vi "Coding_morse3.vi"() -> ()   [LabVIEW 2022 SP3]
panel:
  in  "Alphabet":string[][](array[string])=[["a", ".-"], ["b", "-..."], ["c", "-.-."], ["d", "-.."], ["e", "."], ["f", "..-."], ["g", "--."], ["h", "...."], ["i", ".."], ["j", ".---"], ["k", "-.-"], ["l", ".-.."], ["m", "--"], ["n", "-."], ["o", "---"], ["p", ".--."], ["q", "--.-"], ["r", ".-."], ["s", "..."], ["t", "-"], ["u", "..-"], ["v", "...-"], ["w", ".--"], ["x", "-..-"], ["y", "-.--"], ["z", "--.."], ["1", ".----"], ["2", "..---"], ["3", "...--"], ["4", "....-"], ["5", "....."], ["6", "-...."], ["7", "--..."], ["8", "---.."], ["9", "----."], ["0", "-----"], [" ", "space"]]
  in  "Input Words words":string
  out "Whole code":string[](array[string])
  in  "Dit time(ms)":dbl
  in  "Volume":dbl(knob) scale=0.0..100.0
  in  "Frequency":dbl=500.0
  out "Character code remained":i32
  out "current dit/dash time":dbl
  out "String":string
  out "Current code":string
  out "Waiting until next word":bool
  in  "stop":bool
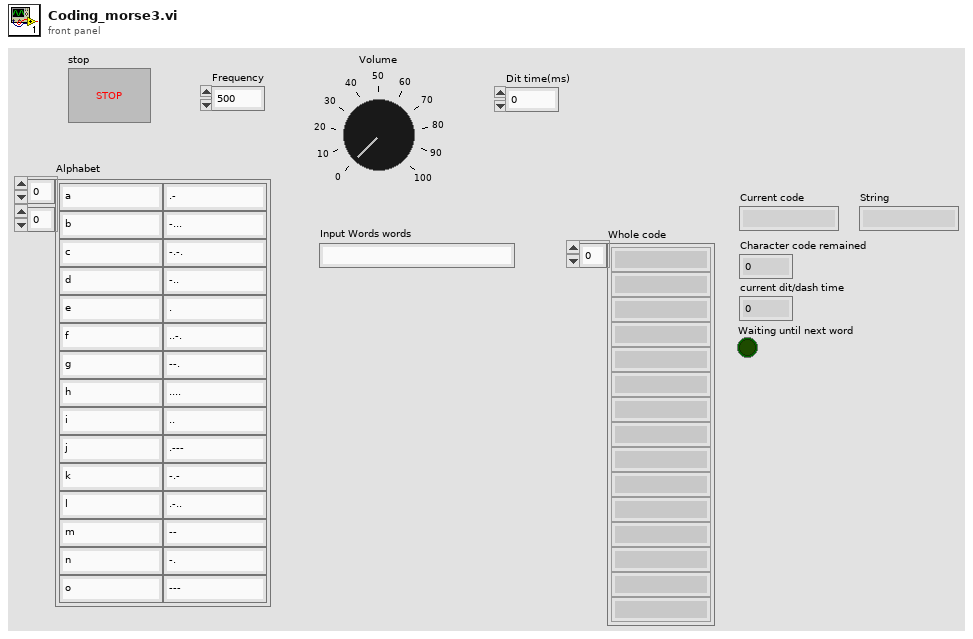
[diagram p1: front panel]
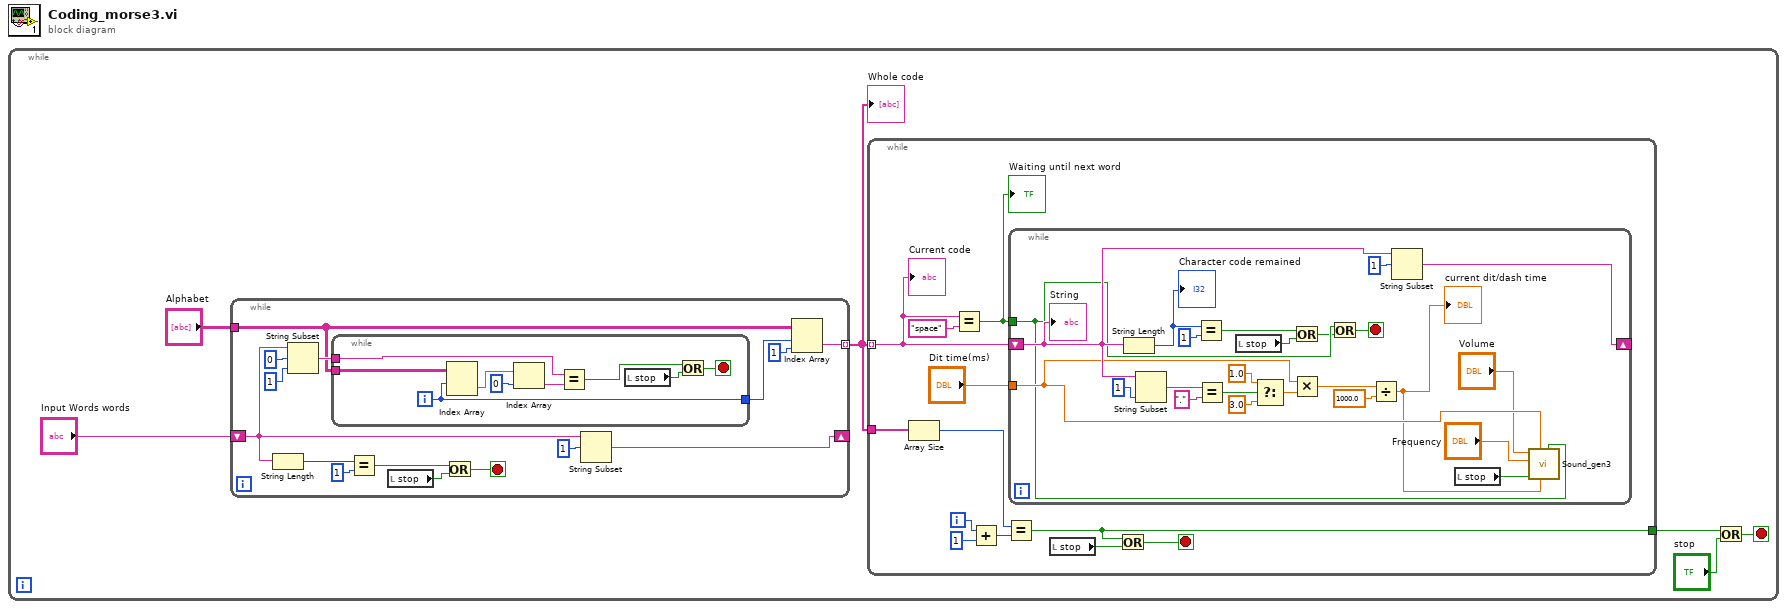
[diagram p0: block diagram]
diagram:
  n1 = while {
    stop <- w1 stop-if-true
    n2 = while {
      shift-right: [w51] -> _
      shift-left: "Input Words words" -> [w52]
      tunnel: "Alphabet" -> [w48]
      tunnel: [w43] -> w4 mode=indexing
      stop <- w44 stop-if-true
      n3 = String Length(string=w52) -> (length=w45:i32)
      n4 = String Subset(string=w52, offset (0)=0, length (rest)=1 ("length (rest)")) -> (substring=w49:string)
      n5 = while {
        tunnel: w48 -> [w66]
        tunnel: w49 -> [w63]
        tunnel: [w58] -> w47
        i -> [w58]
        stop <- w59 stop-if-true
        n6 = Index Array(array=w66, index (row)=w58) -> (element=w64:string[])  [unwired: 1 in]
        n7 = Index Array(array=w64, index=0) -> (element=w62:string)
        n8 = Equal?(x=w63, y=w62) -> (x = y?=w61:bool)
        n9 = local read "stop"() -> (w60:bool)
        n10 = Or(x=w61, y=w60) -> (x .or. y?=w59:bool)
      }
      n11 = Equal?(x=w45, y=1) -> (x = y?=w55:bool)
      n12 = local read "stop"() -> (w56:bool)
      n13 = Or(x=w55, y=w56) -> (x .or. y?=w44:bool)
      n14 = String Subset(string=w52, offset (0)=1) -> (substring=w51:string)  [unwired: 1 in]
      n15 = Index Array(array=w48, index (row)=w47, index (col)=1 ("disabled index (col)")) -> (element=w43:string)
    }
    "Whole code" <- w4
    n16 = while {
      tunnel: w4 -> [w9] mode=indexing
      tunnel: w4 -> [w15]
      tunnel: [w17] -> w3
      i -> [w13]
      stop <- w16 stop-if-true
      n17 = Array Size(array=w15) -> (size(s)=w14:i32)
      n18 = Equal?(x=w9, y="space") -> (x = y?=w7:bool)
      "Waiting until next word" <- w7
      n19 = Add(x=w13, y=1) -> (x+y=w11:i32)
      n20 = Equal?(x=w14, y=w11) -> (x = y?=w17:bool)
      n21 = while {
        shift-right: [w27] -> _
        shift-left: w9 -> [w29]
        tunnel: "Dit time(ms)" -> [w26]
        tunnel: w7 -> [w21]
        stop <- w19 stop-if-true
        n22 = String Length(string=w29) -> (length=w42:i32)
        "Character code remained" <- w42
        n23 = String Subset(string=w29, length (rest)=1 ("length (rest)")) -> (substring=w38:string)  [unwired: 1 in]
        n24 = Equal?(x=w42, y=1) -> (x = y?=w41:bool)
        n25 = Equal?(x=w38, y=".") -> (x = y?=w37:bool)
        n26 = local read "stop"() -> (w40:bool)
        n27 = Select(t=1.0, s=w37, f=3.0) -> (s? t:f=w39:dbl)
        n28 = Or(x=w41, y=w40) -> (x .or. y?=w20:bool)
        n29 = Multiply(x=w26, y=w39) -> (x*y=w32:dbl)
        n30 = Or(x=w21, y=w20) -> (x .or. y?=w19:bool)
        n31 = Divide(x=w32, y=1000.0) -> (x/y=w23:dbl)
        "current dit/dash time" <- w23
        n32 = String Subset(string=w29, offset (0)=1) -> (substring=w27:string)  [unwired: 1 in]
        n33 = local read "stop"() -> (w22:bool)
        n34 = call "Sound_gen3.vi"("Sound/Pause"=w21, "Sound time(s)"=w23, "Dit time(ms)"=w26, "stop"=w22, "Frequency"="Frequency", "Volume"="Volume") -> ()  [unwired: 6 in]
        "String" <- w29
      }
      n35 = local read "stop"() -> (w18:bool)
      n36 = Or(x=w17, y=w18) -> (x .or. y?=w16:bool)
      "Current code" <- w9
    }
    n37 = Or(x=w3, y="stop") -> (x .or. y?=w1:bool)
  }
